vi "Renishaw-XL80_SetUpdateAirCompMethod.vi"(8 "error in (no error)":errorcluster, 11 "Renishaw-XL80_EMU in":refnum<class "Renishaw-XL80_EMU.lvclass">) -> (0 "error out":errorcluster, 3 "Renishaw-XL80_EMU out":refnum<class "Renishaw-XL80_EMU.lvclass">)   [LabVIEW 2024, in "Renishaw-XL80_EMU.lvclass"]
doc: "This method updates the material compensation factor using the most recently acquired material temperature sensor readings.\n\nDefinition\nHRESULTUpdateMatComp();\nParameters\nNone\n\nComments\nThis method will return with an HRESULT of E_FAIL if AutoCompensationMode is set to AUTO_COMPENSATION_FULL. This warns the client that calculating the material compensation factor whilst it is being automatically updated is somewhat pointless.\n\nThis method will also return E_FAIL if the EC10 is disconnected.\n\nIf successful this method will return an HRESULT of S_OK."
uses:
  Renishaw-XL80_EMU.lvclass
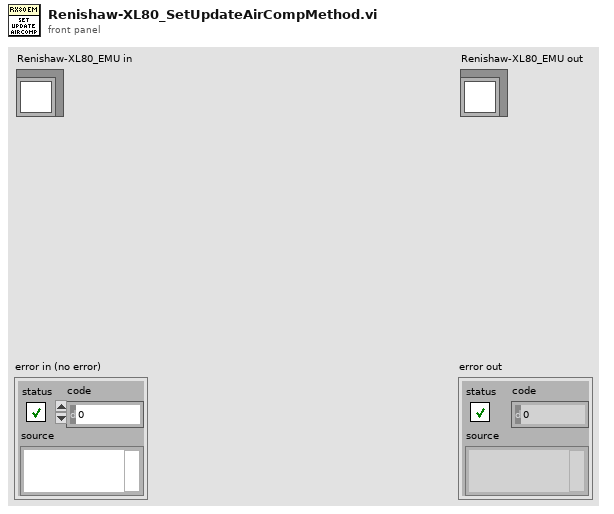
[diagram p1: front panel]
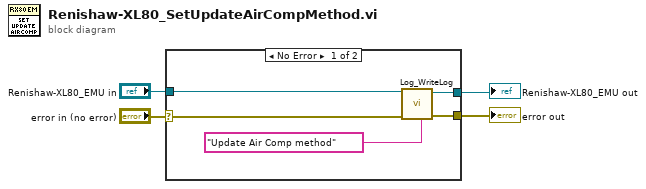
[diagram p0: block diagram]
diagram:
  n1 = case shown="No Error" "error in (no error)" {
    selector: "error in (no error)" -> [w6 w10]
    tunnel: "Renishaw-XL80_EMU in" -> [w9 w11]
    tunnel: [w8 w11] -> w3
    tunnel: [w7 w10] -> w2
    frame No Error {
      n2 = call-dynamic "Log_WriteLog.vi"("Additional text"="Update Air Comp method", "error in (no error)"=w6, "Log in"=w9) -> ("error out"=w7:errorcluster, "Log out"=w8:refnum<class "Renishaw-XL80_EMU.lvclass">)  [unwired: 7 in]
    }
    frame Error {
    }
  }
  "error out" <- w2
  "Renishaw-XL80_EMU out" <- w3
